vi "Extract Input Terminals.vi"(8 "error in (no error)":errorcluster, 11 "Array in":refnum<vi>[](array[refnum])) -> (0 "error out":errorcluster, 1 "description string":string, 2 "names string":string, 3 "Parameter String":string, 4 "defaults string":string, 5 "parameter count":i32, 6 "parameters":string)   [LabVIEW 2025, in "Scripting Server.lvlib"]
uses:
  Scripting Server.lvlib
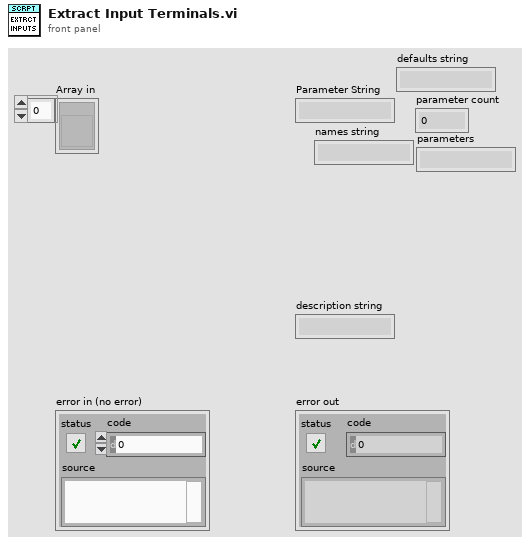
[diagram p1: front panel]
types:
  T1 = typedef "Datatypes.ctl" = enum16{"Float", "Int", "String", "Bool", "Invalid"}
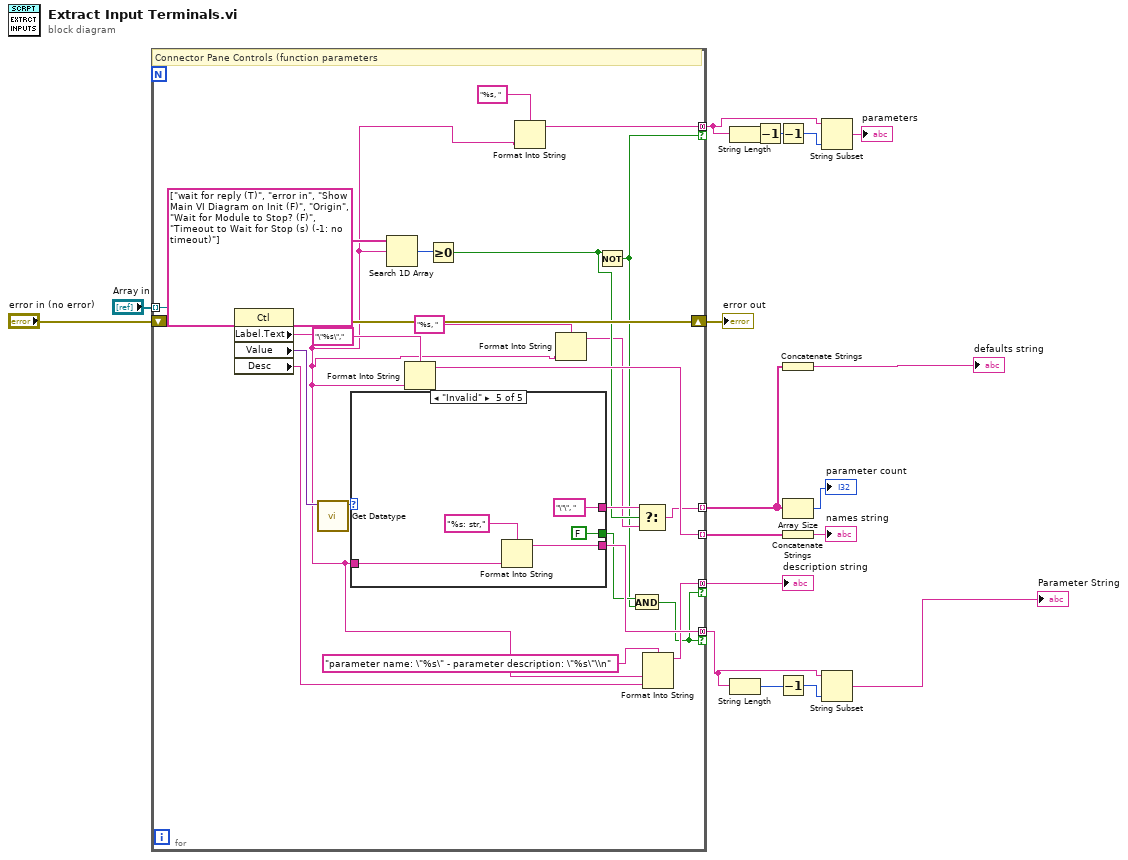
[diagram p0: block diagram]
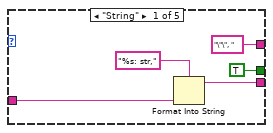
[diagram p2: hidden frame]
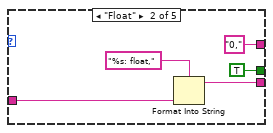
[diagram p3: hidden frame]
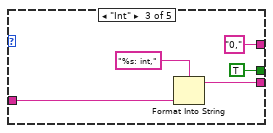
[diagram p4: hidden frame]
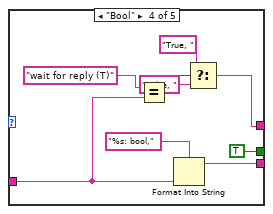
[diagram p5: hidden frame]
diagram:
  n1 = for {
    tunnel: "Array in" -> [w40] mode=indexing
    shift-right: [w41] -> w15
    shift-left: "error in (no error)" -> [w42]
    tunnel: [w38] -> w17 mode=indexing
    tunnel: [w35] -> w7 mode=concatenating if=w27
    tunnel: [w31] -> w18 mode=concatenating if=w27
    tunnel: [w26] -> w11 mode=indexing
    tunnel: [w21] -> w3 mode=concatenating if=w22
    # "Connector Pane Controls (function parameters"
    n2 = property class="Ctl"(reference=w40, error in=w42) -> (error out=w41:errorcluster, "Label.Text"=w20:string, "Value"=w37:variant, "Desc"=w32:string)  [unwired: 1 out]
    n3 = call "Get Datatype.vi"("Value"=w37) -> ("datatypes"=w36:T1)  [unwired: 10 in]
    n4 = case shown="\"Invalid\"" w36 {
      tunnel: w20 -> [w46 w51 w56 w62 w68]
      tunnel: [w45 w50 w55 w65 w67] -> w35
      tunnel: [TRUE TRUE TRUE TRUE FALSE] -> w34
      tunnel: ["\"\", " ("format string") "0," ("format string") "0," ("format string") w59 "\"\", " ("format string")] -> w30
      frame "String" {
        n5 = Format Into String(format string="%s: str,", w46) -> (resulting string=w45:string)  [unwired: 2 in, 1 out]
      }
      frame "Float" {
        n6 = Format Into String(format string="%s: float,", w51) -> (resulting string=w50:string)  [unwired: 2 in, 1 out]
      }
      frame "Int" {
        n7 = Format Into String(format string="%s: int,", w56) -> (resulting string=w55:string)  [unwired: 2 in, 1 out]
      }
      frame "Bool" {
        n8 = Equal?(x="wait for reply (T)" ("String"), y=w62) -> (x = y?=w60:bool)
        n9 = Format Into String(format string="%s: bool,", w62) -> (resulting string=w65:string)  [unwired: 2 in, 1 out]
        n10 = Select(t="True, " ("format string"), s=w60, f="False, ") -> (s? t:f=w59:string)
      }
      frame "Invalid" {
        n11 = Format Into String(format string="%s: str,", w68) -> (resulting string=w67:string)  [unwired: 2 in, 1 out]
      }
    }
    n12 = Search 1D Array(1D array=string[] ["wait for reply (T)", "error in", "Show Main VI Diagram on Init (F)", "Origin", "Wait for Module to Stop? (F)", "Timeout to Wait for Stop (s) (-1: no timeout)"], element=w20) -> (index of element=w28:i32)  [unwired: 1 in]
    n13 = Format Into String(format string="\"%s\",", w20) -> (resulting string=w38:string)  [unwired: 2 in, 1 out]
    n14 = Greater Or Equal To 0?(x=w28) -> (x >= 0?=w25:bool)
    n15 = Format Into String(format string="%s, ", w20) -> (resulting string=w21:string)  [unwired: 2 in, 1 out]
    n16 = Format Into String(format string="%s, ", w20) -> (resulting string=w24:string)  [unwired: 2 in, 1 out]
    n17 = Not(x=w25) -> (.not. x?=w22:bool)
    n18 = And(x=w34, y=w22) -> (x .and. y?=w27:bool)
    n19 = Select(t=w30, s=w25, f=w24) -> (s? t:f=w26:string)
    n20 = Format Into String(format string="parameter name: \"%s\" - parameter description: \"%s\"\\n", w20, w32) -> (resulting string=w31:string)  [unwired: 2 in, 1 out]
  }
  "description string" <- w18
  "error out" <- w15
  n21 = String Length(string=w3) -> (length=w4:i32)
  n22 = String Length(string=w7) -> (length=w9:i32)
  n23 = Decrement(x=w4) -> (x-1=w2:i32)
  n24 = Decrement(x=w2) -> (x-1=w5:i32)
  n25 = Decrement(x=w9) -> (x-1=w8:i32)
  n26 = Concatenate Strings(w11) -> (→"defaults string":string)
  n27 = Array Size(array=w11) -> (size(s)=→"parameter count":i32)
  n28 = Concatenate Strings(w17) -> (→"names string":string)
  n29 = String Subset(string=w3, length (rest)=w5) -> (substring=→"parameters":string)  [unwired: 1 in]
  n30 = String Subset(string=w7, length (rest)=w8) -> (substring=→"Parameter String":string)  [unwired: 1 in]
